vi "Open Pneumatics.vi"(9 "PCM CAN ID":u8) -> ()   [LabVIEW 2018]
uses:
  <vilib>/Rock Robotics/WPI/Solenoid/WPI_SolenoidChannel.ctl
  <vilib>/Rock Robotics/WPI/Solenoid/WPI_SolenoidValue.ctl
  <vilib>/Rock Robotics/WPI/Solenoid/WPI_SolenoidOpenDouble.vi
  <vilib>/Rock Robotics/WPI/Solenoid/WPI_SolenoidOpenSingle.vi
  <vilib>/Rock Robotics/WPI/Utilities/WPI_GetSetVariantRefNum.vi
  <vilib>/Rock Robotics/WPI/Solenoid/WPI_SolenoidSetEnum.vi
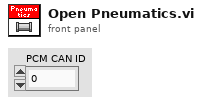
[diagram p1: front panel]
types:
  T1 = typedef "WPI_SolenoidValue.ctl" = enum16{"Off", "On", "Forward", "Reverse"}
  T2 = typedef "WPI_SolenoidChannel.ctl" = enum8{"Solenoid 0", "Solenoid 1", "Solenoid 2", "Solenoid 3", "Solenoid 4", "Solenoid 5", "Solenoid 6", "Solenoid 7", "Invalid"}
  T3 = typedef "WPI_CompressorDevRef.ctl" = cluster{"DevStatus":errorcluster, "Pneumatics Control Module":u8}
  T4 = typedef "WPI_SolenoidDevRef.ctl" = cluster{"DevStatus":errorcluster, "Pneumatics Control Module":u8, "Forward Solenoid Channel":T2, "Reverse Solenoid Channel":T2}
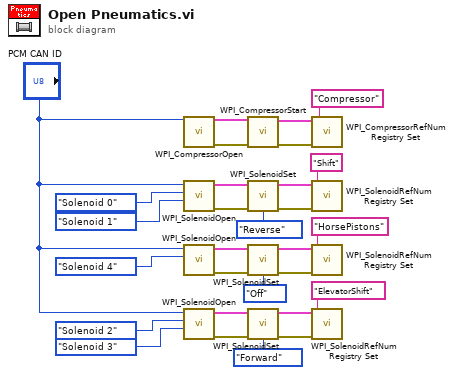
[diagram p0: block diagram]
diagram:
  n1 = call <vilib>:"WPI_CompressorOpen.vi"("Pneumatics Control Module (0)"="PCM CAN ID") -> ("CompressorDevRef"=w27:T3, "error out"=w26:errorcluster)  [unwired: 13 in]
  n2 = call-poly <vilib>:"WPI_SolenoidOpen.vi"("Reverse Solenoid Channel"=WPI_SolenoidChannel."Solenoid 1", "Forward Solenoid Channel"=WPI_SolenoidChannel."Solenoid 0", "Pneumatics Control Module (0)"="PCM CAN ID") -> ("error out"=w9:errorcluster, "SolenoidDevRef"=w15:T4)  [unwired: 7 in]
  n3 = call-poly <vilib>:"WPI_SolenoidOpen.vi"("Solenoid Channel"=WPI_SolenoidChannel."Solenoid 4", "Pneumatics Control Module (0)"="PCM CAN ID") -> ("error out"=w7:errorcluster, "SolenoidDevRef"=w12:T4)  [unwired: 8 in]
  n4 = call-poly <vilib>:"WPI_SolenoidOpen.vi"("Reverse Solenoid Channel"=WPI_SolenoidChannel."Solenoid 3", "Forward Solenoid Channel"=WPI_SolenoidChannel."Solenoid 2" ("Solenoid Channel"), "Pneumatics Control Module (0)"="PCM CAN ID") -> ("error out"=w5:errorcluster, "SolenoidDevRef"=w11:T4)  [unwired: 7 in]
  n5 = call <vilib>:"WPI_CompressorStart.vi"("error in (no error)"=w26, "CompressorDevRef"=w27) -> ("error out"=w29:errorcluster, "CompressorDevRef"=w28:T3)  [unwired: 8 in]
  n6 = call-poly <vilib>:"WPI_SolenoidSet.vi"("error in (no error)"=w9, "Value"=WPI_SolenoidValue."Reverse", "SolenoidDevRef"=w15) -> ("error out"=w8:errorcluster, "SolenoidDevRef"=w14:T4)  [unwired: 7 in]
  n7 = call-poly <vilib>:"WPI_SolenoidSet.vi"("error in (no error)"=w7, "Value"=WPI_SolenoidValue."Off", "SolenoidDevRef"=w12) -> ("error out"=w6:errorcluster, "SolenoidDevRef"=w13:T4)  [unwired: 7 in]
  n8 = call-poly <vilib>:"WPI_SolenoidSet.vi"("error in (no error)"=w5, "Value"=WPI_SolenoidValue."Forward", "SolenoidDevRef"=w11) -> ("error out"=w4:errorcluster, "SolenoidDevRef"=w10:T4)  [unwired: 7 in]
  n9 = call <vilib>:"WPI_CompressorRefNum Registry Set.vi"("error in (no error)"=w29, "refnum name"="Compressor", "CompressorDevRef"=w28) -> ()  [unwired: 7 in, 2 out]
  n10 = call <vilib>:"WPI_SolenoidRefNum Registry Set.vi"("error in (no error)"=w8, "refnum name"="Shift", "SolenoidDevRef"=w14) -> ()  [unwired: 7 in, 2 out]
  n11 = call <vilib>:"WPI_SolenoidRefNum Registry Set.vi"("error in (no error)"=w6, "refnum name"="HorsePistons", "SolenoidDevRef"=w13) -> ()  [unwired: 7 in, 2 out]
  n12 = call <vilib>:"WPI_SolenoidRefNum Registry Set.vi"("error in (no error)"=w4, "refnum name"="ElevatorShift", "SolenoidDevRef"=w10) -> ()  [unwired: 7 in, 2 out]
